vi "Compile and Export Settings.vi"(8 "error in (no error)":errorcluster, 11 "Device Item Ref in":T1 format="%.0x") -> (0 "error out":errorcluster)   [LabVIEW 2019, in "Ghost Bus Addon System Explorer.lvlib"]
uses:
  Ghost Bus Addon System Explorer.lvlib
  <vilib>/NI VeriStand/Custom Device Tools/Custom Device Utility Library/Custom Device Utility Library.lvlib
  Addon Shared/SubVIs/GUID Lookup.vi
  Addon Shared/Ghost Bus Addon Shared.lvlib
  <vilib>/NI VeriStand/Custom Device Tools/Custom Device Utility Library/Search Direction.ctl
  <vilib>/NI VeriStand/Custom Device API/Custom Device API.lvlib
  SubModules/Frame-Protection-Support/Source/Shared/Types/Protection Type.ctl
  SubModules/Frame-Protection-Support/Source/Shared/Protection and Counter Support Shared.lvlib
  SubModules/Frame-Protection-Support/Source/Shared/Types/XNET Signal Configuration.ctl
  <vilib>/NI VeriStand/Custom Device API/Custom Device Item Ref.ctl
  SubModules/Frame-Protection-Support/Source/Shared/Types/Exported Frame Settings.ctl
  SubModules/Frame-Protection-Support/Source/Shared/Types/Exported Counter Settings.ctl
  SubModules/Frame-Protection-Support/Source/Shared/Types/Exported Protection Settings.ctl
  Addon Shared/Types/XNET Settings.ctl
  Addon Shared/Types/Exported.OnCompile.ctl
  <vilib>/NI/NIVS Inline Async API/_Data Access System Explorer/Data Access System Explorer.lvlib
  <vilib>/NI VeriStand/Custom Device Tools/Custom Device Utility Library/NI VeriStand - Search for Item by GUID.vi
  SubModules/Frame-Protection-Support/Source/Shared/Types/Exported Frame Type.ctl
  Addon Shared/Types/986x.ctl
  SubModules/Frame-Protection-Support/Source/System Explorer/Protection and Counter Support System Explorer.lvlib
  SubModules/Frame-Protection-Support/Source/System Explorer/Types/Export Frame GUIDs List.ctl
  SubModules/Frame-Protection-Support/Source/System Explorer/Types/Export Frames List and Type.ctl
  SubModules/Frame-Protection-Support/Source/Shared/Types/Exported Event Trigger Type.ctl
  SubModules/Frame-Protection-Support/Source/System Explorer/Types/Exported Frame Settings.ctl
  <vilib>/NI VeriStand/Custom Device API/Set Item Property (Variant).vi
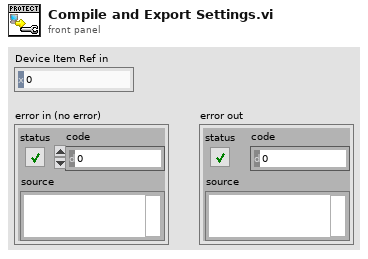
[diagram p1: front panel]
types:
  T1 = typedef "Custom Device API.lvlib/Custom Device Item Ref.ctl" = u64
  T2 = cluster{"Name":string, "Type":enum16{"Output/Write", "Input/Read", "Input/ReadWrite"}, "VS Refs":T1[]}
  T3 = typedef "Protection and Counter Support System Explorer.lvlib/Export Frames List and Type.ctl" = cluster{"Type":T4, "Frame Refs":T1[], "Frame Settings":T5[]}
  T4 = typedef "Protection and Counter Support Shared.lvlib/Exported Frame Type.ctl" = enum16{"Periodic", "Event", "Periodic/Event"}
  T5 = typedef "Protection and Counter Support System Explorer.lvlib/Exported Frame Settings.ctl" = cluster{"ID":u32, "Disable Transmission":bool, "Disable Transmission Ref":T1, "Transmit Trigger":T6, "Transmit Trigger Ref":T1}
  T6 = typedef "Protection and Counter Support Shared.lvlib/Exported Event Trigger Type.ctl" = enum16{"Channel value change", "Trigger channel (not zero)", "Channel value change or trigger channel (not zero)", "Trigger channel (any value change)", "Channel value change or trigger channel (any value change)"}
  T7 = typedef "Custom Device Utility Library.lvlib/Search Direction.ctl" = enum16{"Down", "Up"}
  T8 = typedef "Protection and Counter Support System Explorer.lvlib/Export Frame GUIDs List.ctl" = cluster{"Signal Page GUID":string, "Rolling Counter Value GUID":string, "Protection Value GUID":string, "Time Difference GUID":string, "Receive Time GUID":string}
  T9 = typedef "Ghost Bus Addon Shared.lvlib/Exported.OnCompile.ctl" = cluster{"Name":string, "XNET Settings":T10, "Frames":T11[], "986x Support":T16, "Incoming Frames":T11[]}
  T10 = typedef "Ghost Bus Addon Shared.lvlib/XNET Settings.ctl" = cluster{"Database":refnum<k21>, "Cluster":refnum<k21>, "Port":string, "Baud rate [Bd]":u64, "Termination":u32, "CAN I/O Mode":u32, "FD Baud rate [Bd]":u64, "Priority":i32, "Use Legacy":bool, "FD ISO Mode":u32}
  T11 = typedef "Protection and Counter Support Shared.lvlib/Exported Frame Settings.ctl" = cluster{"Type":T4, "Frame ID":u32, "Payload Length":u32, "Signal XNET Paths":string[], "Frame.PrevData":dbl[], "VS Offset":i32, "VS Length":i32, "Generation Period":u32, "Has Protection?":bool, "Protection Configurations":T12[], "Has Counter":bool, "Counter Configurations":T15[], "Has Disable?":bool, "Disable VS Index":i32, "Transmit Trigger":T6, "Trigger VS Index":i32}
  T12 = typedef "Protection and Counter Support Shared.lvlib/Exported Protection Settings.ctl" = cluster{"Protection Frame Index":i32, "Protection Type":T13, "Data Indeces":i32[], "Initialized Data Array":dbl[], "Protection Signal XNET Paths":string[], "CRC Channels":T14[], "Protection VS Update Index":i32, "Override Index":i32, "Override Value Index":i32}
  T13 = typedef "Protection and Counter Support Shared.lvlib/Protection Type.ctl" = enum16{"Arb ID + Bytes Checksum with Inversion", "Arb ID + Bytes CRC with Inversion", "Reversed Raw Signal Checksum with Inversion", "Concatenated Two's Compliment"}
  T14 = typedef "Protection and Counter Support Shared.lvlib/XNET Signal Configuration.ctl" = cluster{"Start Bit":i32, "Name":string, "Number of bits":i32, "Scale":dbl, "Offset":dbl, "Data Type":u32, "Counter":bool}
  T15 = typedef "Protection and Counter Support Shared.lvlib/Exported Counter Settings.ctl" = cluster{"Frame Index":i32, "Max Count":dbl, "VS Index":i32, "Bit Length":i64, "Override Index":i32, "Override Value Index":i32}
  T16 = typedef "Ghost Bus Addon Shared.lvlib/986x.ctl" = cluster{"Enable":bool, "RIO Device":string, "Bitfile":path}
  T17 = typedef "Custom Device API.lvlib/Custom Device Item Info.ctl" = cluster{"Name":string, "Is Channel":bool, "GUID":string, "Is Waveform":bool}
  T18 = typedef "Protection and Counter Addon Shared.lvlib/986x.ctl" = cluster{"Enable":bool, "RIO Device":string, "Bitfile":path}
  T19 = typedef "Ghost Bus Addon System Explorer.lvlib/Frame Settings.ctl" = cluster{"ID":u32, "Disable Transmission":bool, "Disable Transmission Ref":T1, "Transmit Trigger":T20, "Transmit Trigger Ref":T1}
  T20 = typedef "Ghost Bus Addon System Explorer.lvlib/Event Trigger Type.ctl" = enum16{"Channel value change", "Trigger channel (not zero)", "Channel value change or trigger channel (not zero)", "Trigger channel (any value change)", "Channel value change or trigger channel (any value change)"}
  T21 = cluster{"Name":string, "Type":enum16{"Output/Write", "Input/Read", "Input/ReadWrite"}, "VS Refs":T1[]}[]
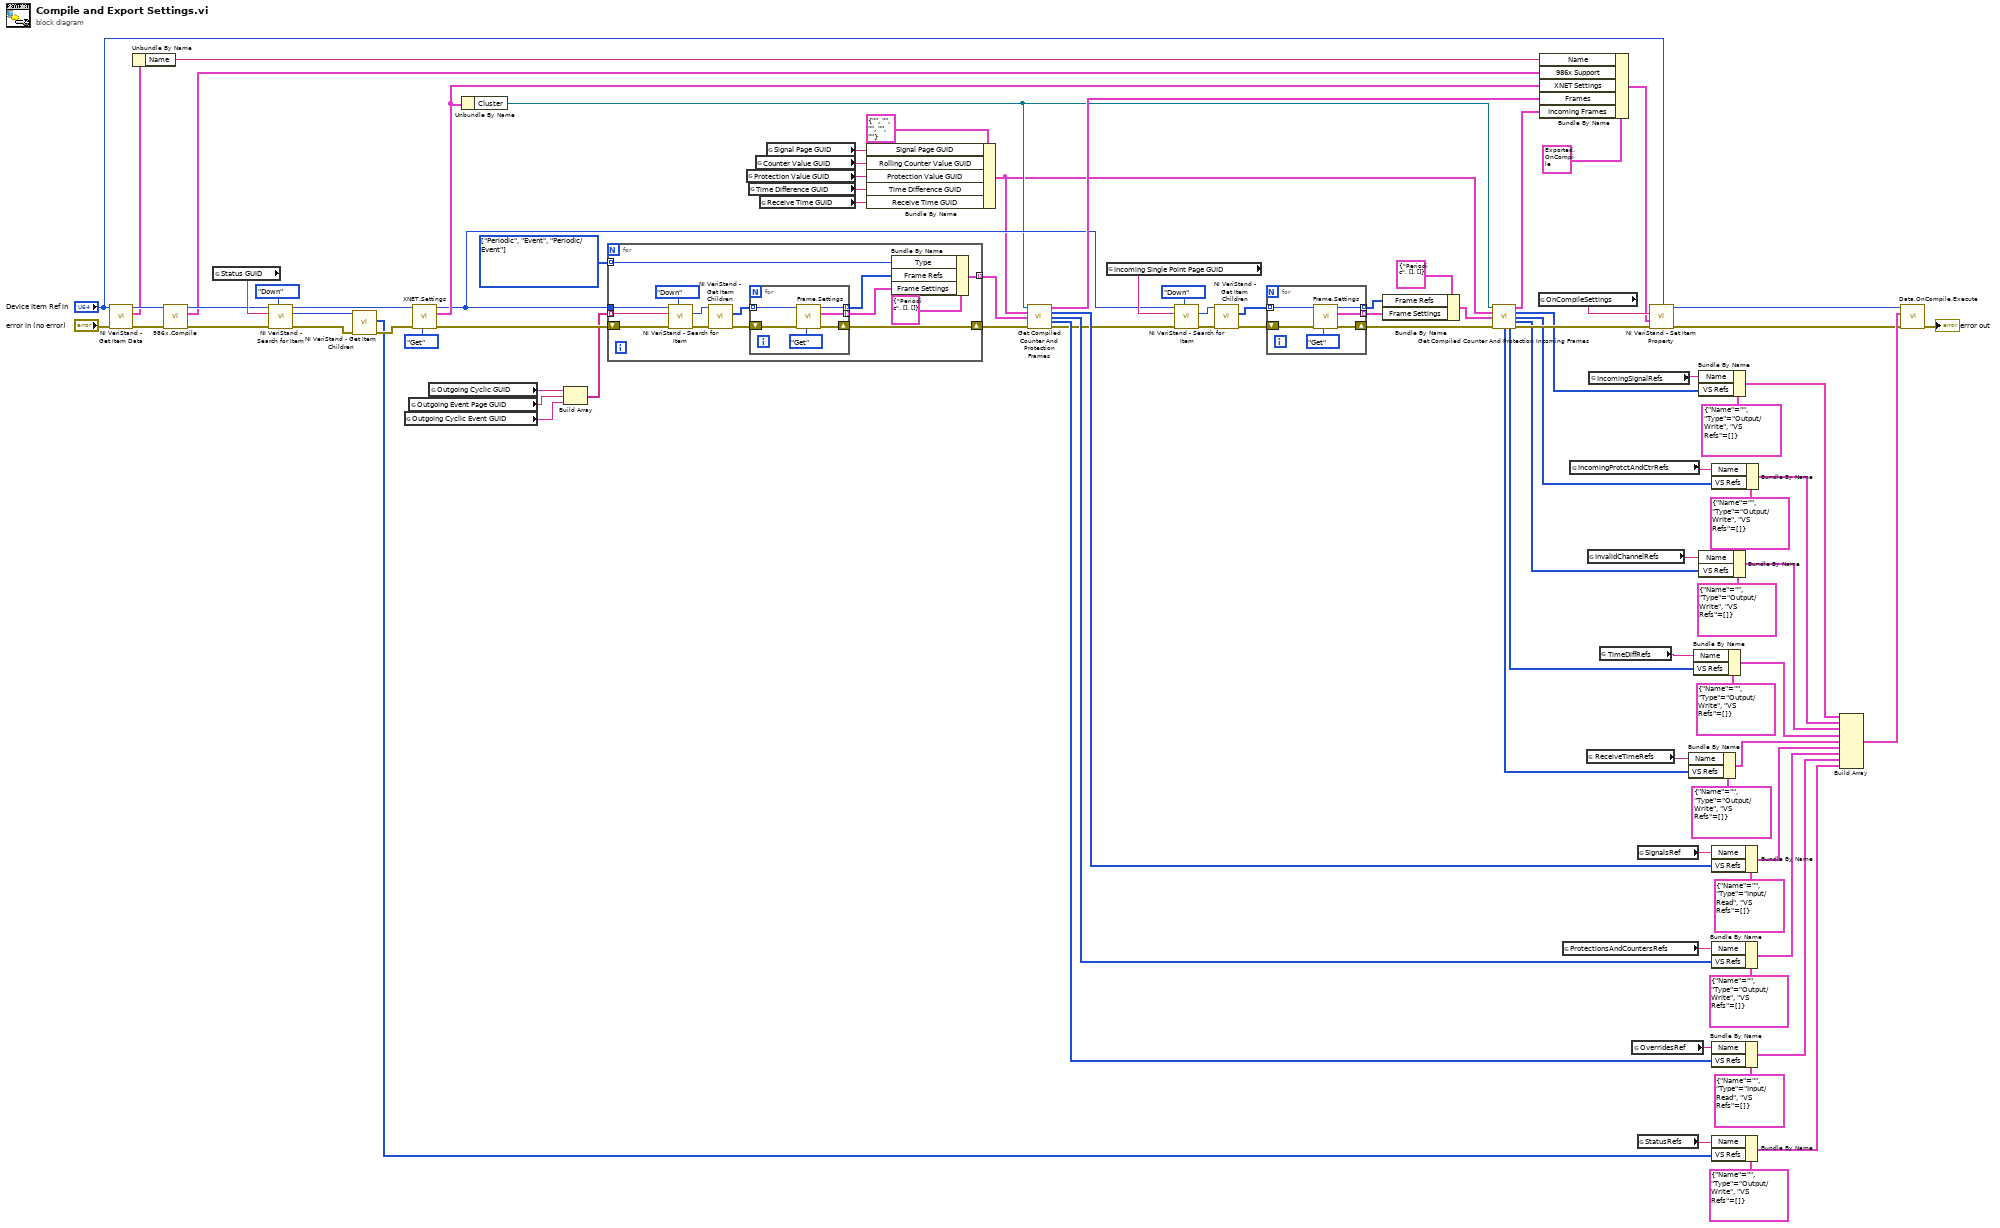
[diagram p0: block diagram]
diagram:
  w61 = T4[] [enum."Periodic", enum."Event", enum."Periodic/Event"] items=["Periodic", "Event", "Periodic/Event"]
  n1 = call <vilib>:"NI VeriStand - Get Item Data.vi"("error in (no error)"="error in (no error)", "Item Ref in"="Device Item Ref in") -> ("error out"=w48:errorcluster, "Item Info"=w46:T17, "Item Ref out"=w47:T1)  [unwired: 6 in, 1 out]
  n2 = Unbundle By Name(w46) -> ("Name"=w45:string)
  n3 = call "986x.Compile.vi"("error in (no error)"=w48, "Item Ref in"=w47) -> ("error out"=w68:errorcluster, "986x Support"=w58:T18, "Item Ref out"=w67:T1)  [unwired: 7 in]
  n4 = global read "GUID Lookup.vi" "Status GUID"() -> (w75:string)
  n5 = call-poly <vilib>:"NI VeriStand - Search for Item.vi"("Direction (Down)"=Search_Direction."Down", "error in"=w68, "Item GUID"=w75, "Section Ref in"=w67) -> ("error out"=w72:errorcluster, "Item Ref"=w73:T1, "Section Ref out"=w74:T1)  [unwired: 4 in, 1 out]
  n6 = call <vilib>:"NI VeriStand - Get Item Children.vi"("error in (no error)"=w72, "Item Ref in"=w73) -> ("error out"=w71:errorcluster, "Child Refs"=w70:T1[])  [unwired: 6 in, 2 out]
  n7 = global read "GUID Lookup.vi" "Outgoing Cyclic Event GUID"() -> (w53:string)
  n8 = global read "GUID Lookup.vi" "Outgoing Event Page GUID"() -> (w54:string)
  n9 = call "XNET.Settings.vi"("Action"=enum8{"Get", "Set"}."Get", "error in (no error)"=w71, "Parent Ref in"=w74) -> ("error out"=w52:errorcluster, "XNET Settings"=w90:T10, "Item Ref out"=w32:T1)  [unwired: 6 in]
  n10 = global read "GUID Lookup.vi" "Outgoing Cyclic GUID"() -> (w55:string)
  n11 = Unbundle By Name(w90) -> ("Cluster"=w15:refnum<k21>)
  n12 = Build Array(w55, w54, w53) -> (w51:string[])
  n13 = for {
    shift-right: [w93] -> w62
    shift-left: w52 -> [w103]
    tunnel: w61 -> [w106] mode=indexing
    tunnel: [w105] -> w60 mode=indexing
    tunnel: w32 -> [w102]
    tunnel: w51 -> [w101] mode=indexing
    n14 = call-poly <vilib>:"NI VeriStand - Search for Item.vi"("Direction (Down)"=Search_Direction."Down", "error in"=w103, "Item GUID"=w101, "Section Ref in"=w102) -> ("error out"=w99:errorcluster, "Item Ref"=w100:T1)  [unwired: 4 in, 2 out]
    n15 = call <vilib>:"NI VeriStand - Get Item Children.vi"("error in (no error)"=w99, "Item Ref in"=w100) -> ("error out"=w97:errorcluster, "Child Refs"=w96:T1[])  [unwired: 6 in, 2 out]
    n16 = for {
      tunnel: w96 -> [w110] mode=indexing
      shift-right: [w109] -> w93
      shift-left: w97 -> [w111]
      tunnel: [w108] -> w95 mode=indexing
      tunnel: [w107] -> w94 mode=indexing
      n17 = call "Frame.Settings.vi"("Action"=enum8{"Get", "Set"}."Get", "error in (no error)"=w111, "Item Ref in"=w110) -> ("error out"=w109:errorcluster, "Frame.Settings"=w107:T19, "Item Ref out"=w108:T1)  [unwired: 6 in]
    }
    n18 = Bundle By Name(cluster=T3 {"Type"=enum."Periodic", "Frame Refs"=[], "Frame Settings"=[]} ("Export Frames List and Type"), "Type"=w106, "Frame Refs"=w95, "Frame Settings"=w94) -> (w105:T3)
  }
  n19 = global read "GUID Lookup.vi" "Protection Value GUID"() -> (w64:string)
  n20 = global read "GUID Lookup.vi" "Time Difference GUID"() -> (w2:string)
  n21 = global read "GUID Lookup.vi" "Counter Value GUID"() -> (w65:string)
  n22 = global read "GUID Lookup.vi" "Receive Time GUID"() -> (w1:string)
  n23 = global read "GUID Lookup.vi" "Signal Page GUID"() -> (w66:string)
  n24 = Bundle By Name(cluster=T8 {"Signal Page GUID"="", "Rolling Counter Value GUID"="", "Protection Value GUID"="", "Time Difference GUID"="", "Receive Time GUID"=""}, "Signal Page GUID"=w66, "Rolling Counter Value GUID"=w65, "Protection Value GUID"=w64, "Time Difference GUID"=w2, "Receive Time GUID"=w1) -> (w14:T8)
  n25 = call "Get Compiled Counter And Protection Frames.vi"("XNET Cluster"=w15, "GUIDs"=w14, "Frames per type"=w60, "error in (no error)"=w62) -> ("Frames"=w56:T11[], "Signals Refs"=w57:T1[], "Counters and Protection Refs"=w85:T1[], "Override Refs"=w41:T1[], "error out"=w37:errorcluster)  [unwired: 7 in]
  n26 = global read "GUID Lookup.vi" "Incoming Single Point Page GUID"() -> (w36:string)
  n27 = call-poly <vilib>:"NI VeriStand - Search for Item.vi"("Direction (Down)"=Search_Direction."Down", "error in"=w37, "Item GUID"=w36, "Section Ref in"=w32) -> ("error out"=w38:errorcluster, "Item Ref"=w39:T1)  [unwired: 4 in, 2 out]
  n28 = call <vilib>:"NI VeriStand - Get Item Children.vi"("error in (no error)"=w38, "Item Ref in"=w39) -> ("error out"=w35:errorcluster, "Child Refs"=w33:T1[])  [unwired: 6 in, 2 out]
  n29 = for {
    tunnel: w33 -> [w116] mode=indexing
    shift-right: [w115] -> w34
    shift-left: w35 -> [w117]
    tunnel: [w114] -> w30 mode=indexing
    tunnel: [w113] -> w29 mode=indexing
    n30 = call "Frame.Settings.vi"("Action"=enum8{"Get", "Set"}."Get", "error in (no error)"=w117, "Item Ref in"=w116) -> ("error out"=w115:errorcluster, "Frame.Settings"=w113:T19, "Item Ref out"=w114:T1)  [unwired: 6 in]
  }
  n31 = Bundle By Name(cluster=T3 {"Type"=enum."Periodic", "Frame Refs"=[], "Frame Settings"=[]} ("Export Frames List and Type"), "Frame Refs"=w30, "Frame Settings"=w29) -> (w13:T3)
  n32 = call "Get Compiled Counter And Protection Incoming Frames.vi"("XNET Cluster"=w15, "GUIDs"=w14, "Incoming Frames In"=w13, "error in (no error)"=w34) -> ("Incoming Frames Out"=w12:T11[], "Signals Refs"=w11:T1[], "Counters and Protection Refs"=w10:T1[], "Invalid Refs"=w9:T1[], "Rcv Time Refs"=w7:T1[], "Time Diff Refs"=w8:T1[], "error out"=w16:errorcluster)  [unwired: 5 in]
  n33 = global read "GUID Lookup.vi" "OnCompileSettings"() -> (w80:string)
  n34 = Bundle By Name(cluster=T9 {"Name"="", "XNET Settings"={"Database"="", "Cluster"="", "Port"="", "Baud rate [Bd]"=500000, "Termination"=1, "CAN I/O Mode"=0, "FD Baud rate [Bd]"=500000, "Priority"=100, "Use Legacy"=FALSE, "FD ISO Mode"=0}, "Frames"=[], "986x Support"={"Enable"=FALSE, "RIO Device"="", "Bitfile"=path ""}, "Incoming Frames"=[]}, "Name"=w45, "986x Support"=w58, "XNET Settings"=w90, "Frames"=w56, "Incoming Frames"=w12) -> (w21:T9)
  n35 = global read "GUID Lookup.vi" "ProtectionsAndCountersRefs"() -> (w81:string)
  n36 = global read "GUID Lookup.vi" "IncomingProtctAndCtrRefs"() -> (w17:string)
  n37 = global read "GUID Lookup.vi" "ReceiveTimeRefs"() -> (w24:string)
  n38 = global read "GUID Lookup.vi" "InvalidChannelRefs"() -> (w25:string)
  n39 = global read "GUID Lookup.vi" "IncomingSignalRefs"() -> (w26:string)
  n40 = global read "GUID Lookup.vi" "TimeDiffRefs"() -> (w20:string)
  n41 = global read "GUID Lookup.vi" "OverridesRef"() -> (w44:string)
  n42 = global read "GUID Lookup.vi" "SignalsRef"() -> (w82:string)
  n43 = global read "GUID Lookup.vi" "StatusRefs"() -> (w77:string)
  n44 = call-poly <vilib>:"NI VeriStand - Set Item Property.vi"("error in (no error)"=w16, "Value"=w21, "Property Name"=w80, "Item Ref in"="Device Item Ref in") -> ("error out"=w84:errorcluster, "Item Ref out"=w83:T1)  [unwired: 5 in, 1 out]
  n45 = Bundle By Name(cluster=T2 {"Name"="", "Type"=enum."Output/Write", "VS Refs"=[]} ("Group"), "Name"=w24, "VS Refs"=w7) -> (w3:T2)
  n46 = Bundle By Name(cluster=T2 {"Name"="", "Type"=enum."Output/Write", "VS Refs"=[]} ("Group"), "Name"=w20, "VS Refs"=w8) -> (w4:T2)
  n47 = Bundle By Name(cluster=T2 {"Name"="", "Type"=enum."Output/Write", "VS Refs"=[]} ("Group"), "Name"=w26, "VS Refs"=w11) -> (w22:T2)
  n48 = Bundle By Name(cluster=T2 {"Name"="", "Type"=enum."Output/Write", "VS Refs"=[]} ("Group"), "Name"=w25, "VS Refs"=w9) -> (w5:T2)
  n49 = Bundle By Name(cluster=T2 {"Name"="", "Type"=enum."Input/Read", "VS Refs"=[]} ("Group"), "Name"=w82, "VS Refs"=w57) -> (w88:T2)
  n50 = Bundle By Name(cluster=T2 {"Name"="", "Type"=enum."Output/Write", "VS Refs"=[]} ("Group"), "Name"=w81, "VS Refs"=w85) -> (w79:T2)
  n51 = Bundle By Name(cluster=T2 {"Name"="", "Type"=enum."Input/Read", "VS Refs"=[]} ("Group"), "Name"=w44, "VS Refs"=w41) -> (w42:T2)
  n52 = Bundle By Name(cluster=T2 {"Name"="", "Type"=enum."Output/Write", "VS Refs"=[]} ("Group"), "Name"=w77, "VS Refs"=w70) -> (w59:T2)
  n53 = Bundle By Name(cluster=T2 {"Name"="", "Type"=enum."Output/Write", "VS Refs"=[]} ("Group"), "Name"=w17, "VS Refs"=w10) -> (w6:T2)
  n54 = Build Array(w22, w6, w5, w4, w3, w88, w79, w42, w59) -> (w87:T21)
  n55 = call <vilib>:"Data.OnCompile.Execute.vi"("error in"=w84, "VS Ref Groups"=w87, "Custom Device Ref"=w83) -> ("error out"=→"error out":errorcluster)  [unwired: 7 in, 1 out]
